vi "NurseStationMain.vi"() -> ()   [LabVIEW 2015]
uses:
  TypeDef/SelectedRoom.ctl
  TypeDef/ColorFlags.ctl
  Classes/Room/Room.lvclass/Room.ctl
  TypeDef/State Cluster.ctl
  Classes/Room/Room.lvclass
  Classes/Room/Read Flags.lvclass.vi
  Classes/Flags/Flags.lvclass
panel:
  in  "stop":bool
  in  "Tab Control":enum32{"Main View", "Reports"}(tab)
  out "Rooms":T1[](array[typedef])
  out "Selected Room":T2={"RoomNumFlags"={"Room Number"=0, "Flag State"=[1, 3, 5, 7]}, "BedVacant"=FALSE, "InRoomPersonnel"=[], "RoomRequests"=[]}
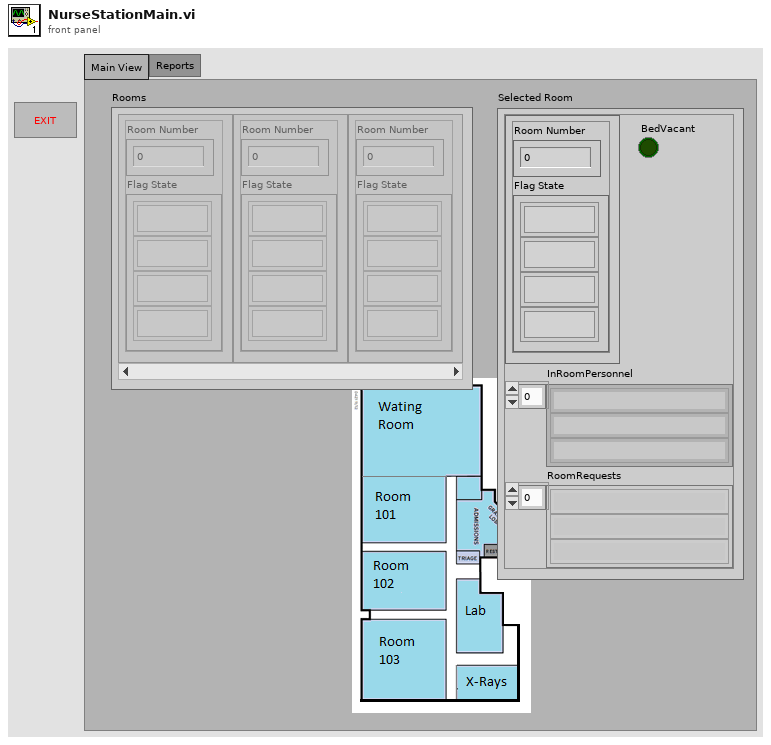
[diagram p1: front panel]
types:
  T1 = typedef "ColorFlags.ctl" = cluster{"Room Number":u32, "Flag State":u8[]}
  T2 = typedef "SelectedRoom.ctl" = cluster{"RoomNumFlags":cluster{"Room Number":u8, "Flag State":u8[]}, "BedVacant":bool, "InRoomPersonnel":string[], "RoomRequests":string[]}
  T3 = typedef "EventsReference.ctl" = cluster{"Init":refnum<user-event>, "Refresh UI":refnum<user-event>}
  T4 = typedef "State Cluster.ctl" = cluster{"Room Array":refnum<class "Room.lvclass">[], "Selected Room":u32}
  T5 = typedef "LVPoint32TypeDef.ctl" = cluster{"Horizontal":i32, "Vertical":i32}
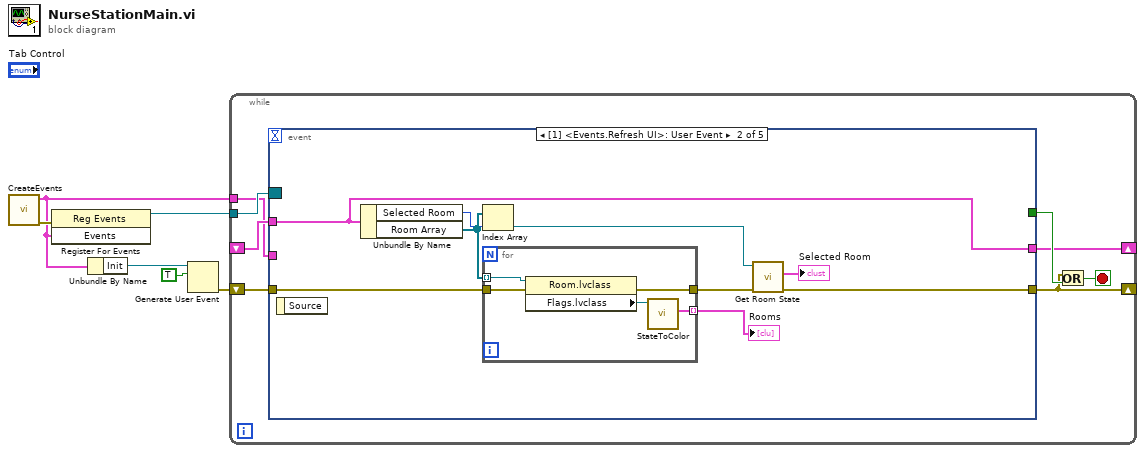
[diagram p0: block diagram]
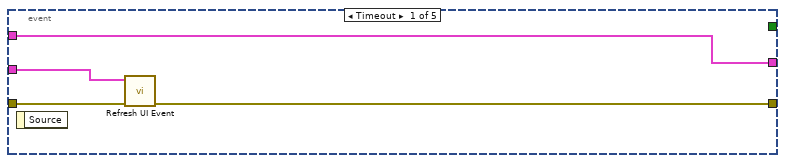
[diagram p2: hidden frame]
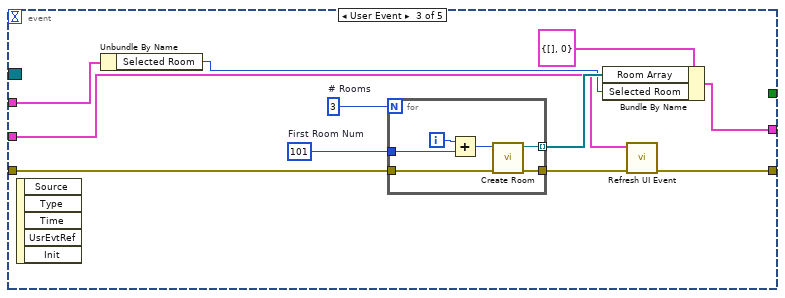
[diagram p3: hidden frame]
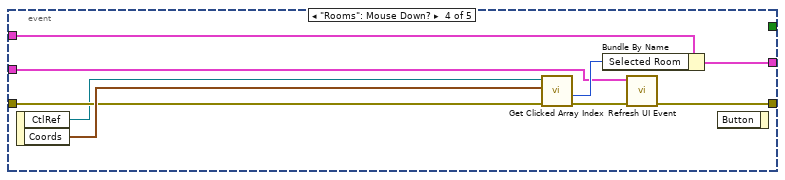
[diagram p4: hidden frame]
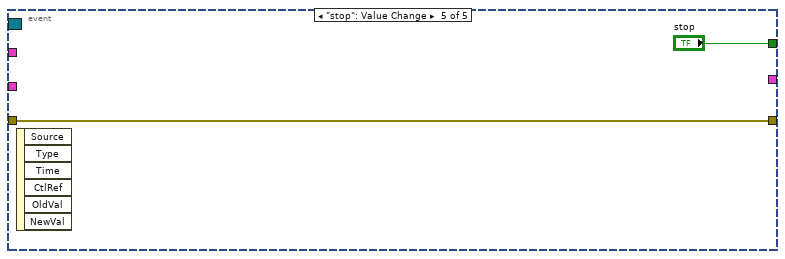
[diagram p5: hidden frame]
diagram:
  n1 = call "CreateEvents.vi"() -> ("error out"=w6:errorcluster, "Events"=w2:T3)  [unwired: 10 in]
  n2 = register-events(error in=w6, w2) -> (reference out=w5:refnum<event-registration>)  [unwired: 1 in, 1 out]
  n3 = Unbundle By Name(w2) -> ("Init"=w4:refnum<user-event>)
  n4 = Generate User Event(user event=w4, event data cluster=TRUE ("event data")) -> (error out=w1:errorcluster)  [unwired: 2 in, 1 out]
  n5 = while {
    shift-right: [w8] -> _
    shift-left: _ -> [w9]
    shift-right: [w11] -> _
    shift-left: w1 -> [w14]
    tunnel: w5 -> [w10]
    tunnel: w2 -> [w7]
    stop <- w12 stop-if-true
    n6 = event shown="[1] <Events.Refresh UI>: User Event" {
      selector: w10 -> [_ _ _ _ _]
      dyn-events: _ -> [_ _ _ _ _]
      timeout: _ -> [_ _ _ _ _]
      tunnel: w14 -> [w17 w23 w35 w57 w59]
      tunnel: [w16 w21 w36 w51 w59] -> w11
      tunnel: [_ _ _ _ "stop"] -> w13
      tunnel: w9 -> [w15 w26 w34 w56 _]
      tunnel: [w15 w26 w40 w55 _] -> w8
      tunnel: w7 -> [w18 _ w38 w53 _]
      event Timeout {
        n7 = event-data() -> ()  [unwired: 1 in, 1 out]
        n8 = call "Refresh UI Event.vi"("error in (no error)"=w17, "Events"=w18) -> ("error out"=w16:errorcluster)  [unwired: 9 in]
      }
      event User Event {
        n9 = event-data() -> ()  [unwired: 1 in, 1 out]
        n10 = Unbundle By Name(w26) -> ("Selected Room"=w24:u32, "Room Array"=w25:refnum<class "Room.lvclass">[])
        n11 = Index Array(array=w25, index=w24) -> (element=w19:refnum<class "Room.lvclass">)
        n12 = for {
          tunnel: [w31] -> w27 mode=indexing
          tunnel: w25 -> [w30] mode=indexing
          tunnel: w23 -> [w29]
          tunnel: [w28] -> w22
          n13 = property class="Room.lvclass"(reference=w30, error in=w29) -> (error out=w28:errorcluster, "Flags.lvclass"=w32:refnum<class "Flags.lvclass">)  [unwired: 1 out]
          n14 = call "StateToColor.vi"("Flags in"=w32) -> ("RoomNumFlags"=w31:T1)  [unwired: 8 in, 2 out]
        }
        "Rooms" <- w27
        n15 = call "Get Room State.vi"("error in"=w22, "Room In"=w19) -> ("error out"=w21:errorcluster, "Selected Room"=→"Selected Room":T2)  [unwired: 7 in, 1 out]
      }
      event User Event {
        w42 = 3  # # Rooms
        w43 = u32 101  # First Room Num
        n16 = event-data() -> ()  [unwired: 1 in, 5 out]
        n17 = Unbundle By Name(w34) -> ("Selected Room"=w33:u32)
        n18 = for {
          N: w42 -> [_]
          tunnel: w43 -> [w49]
          tunnel: [w48] -> w37
          tunnel: [w47] -> w41 mode=indexing
          tunnel: w35 -> [w44]
          i -> [w45]
          n19 = Add(x=w45, y=w49) -> (x+y=w46:u32)
          n20 = call "Create Room.vi"("error in"=w44, "Room Number"=w46) -> ("error out"=w48:errorcluster, "Room Ref"=w47:refnum<class "Room.lvclass">)  [unwired: 8 in]
        }
        n21 = Bundle By Name(cluster=T4 {"Room Array"=[], "Selected Room"=0} ("State Cluster"), "Room Array"=w41, "Selected Room"=w33) -> (w40:T4)
        n22 = call "Refresh UI Event.vi"("error in (no error)"=w37, "Events"=w38) -> ("error out"=w36:errorcluster)  [unwired: 9 in]
      }
      event "Rooms": Mouse Down? {
        n23 = event-data() -> ("CtlRef"=w50:refnum<vi>, "Coords"=w58:T5)  [unwired: 1 in]
        n24 = call "Get Clicked Array Index.vi"("error in"=w57, "Coordinates"=w58, "CtlRef"=w50) -> ("error out"=w52:errorcluster, "Column"=w54:i32)  [unwired: 6 in, 1 out]
        n25 = Bundle By Name(cluster=w56, "Selected Room"=w54) -> (w55:T4)
        n26 = call "Refresh UI Event.vi"("error in (no error)"=w52, "Events"=w53) -> ("error out"=w51:errorcluster)  [unwired: 9 in]
        n27 = event-data() -> ()  [unwired: 2 in, 1 out]
      }
      event "stop": Value Change {
        n28 = event-data() -> ()  [unwired: 1 in, 6 out]
      }
    }
    n29 = Or(x=w11, y=w13) -> (x .or. y?=w12:bool)
  }
